vi "Save MC Test Data.vi"(5 "Initialise":bool, 6 "Stop":bool, 7 "Actual refresh rate (ms)":u32, 8 "error in (no error)":errorcluster, 9 "Initial Time Stamp":timestamp, 10 "Test Data In":dbl[][](array[numeric]), 11 "FPGA Ref in":T1) -> (0 "error out":errorcluster, 1 "MC state":enum16{"Waiting", "First frame", "Wrote Ref"}(ring), 2 "Test Data Out":dbl[][](array[numeric]), 4 "MC Data Save ON":bool)   [LabVIEW 2020]
uses:
  RIG-SPECIFIC FILES/FPGA Refs/FPGA Ref.ctl
  <vilib>/Utility/error.llb/Error Cluster From Error Code.vi
  <vilib>/rvi/errors/niLvFpgaAdjustHostInterfaceError.vi
  <vilib>/rvi/interface/nirviReadWriteControl/nirviReadWriteControl.xnode
  NiFpgaLv.dll
  <vilib>/rvi/interface/Simulation/niFpgaSimulationCallBeginRW.vi
panel:
  out "num_xyref_pixels":u16
  out "numxyzpixels":u16
  out "y_offset 3":fxp<+/-,16,8>
  out "X_Y_Z":bool[](array[boolean])
  out "MC state 2":enum16{"Waiting", "First frame", "Wrote Ref"}(ring)
  out "y_offset 2":fxp<+/-,16,8>
  out "y_offset":fxp<+/-,16,8>
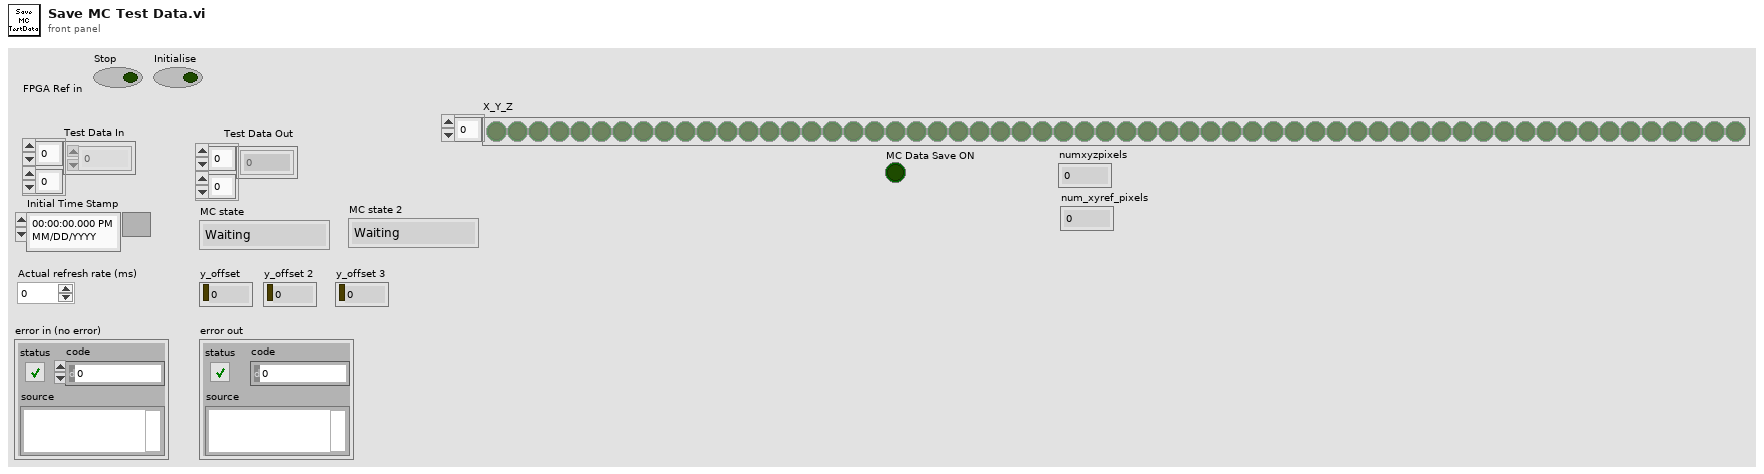
[diagram p1: front panel]
types:
  T1 = typedef "FPGA Ref.ctl" = refnum<k20>
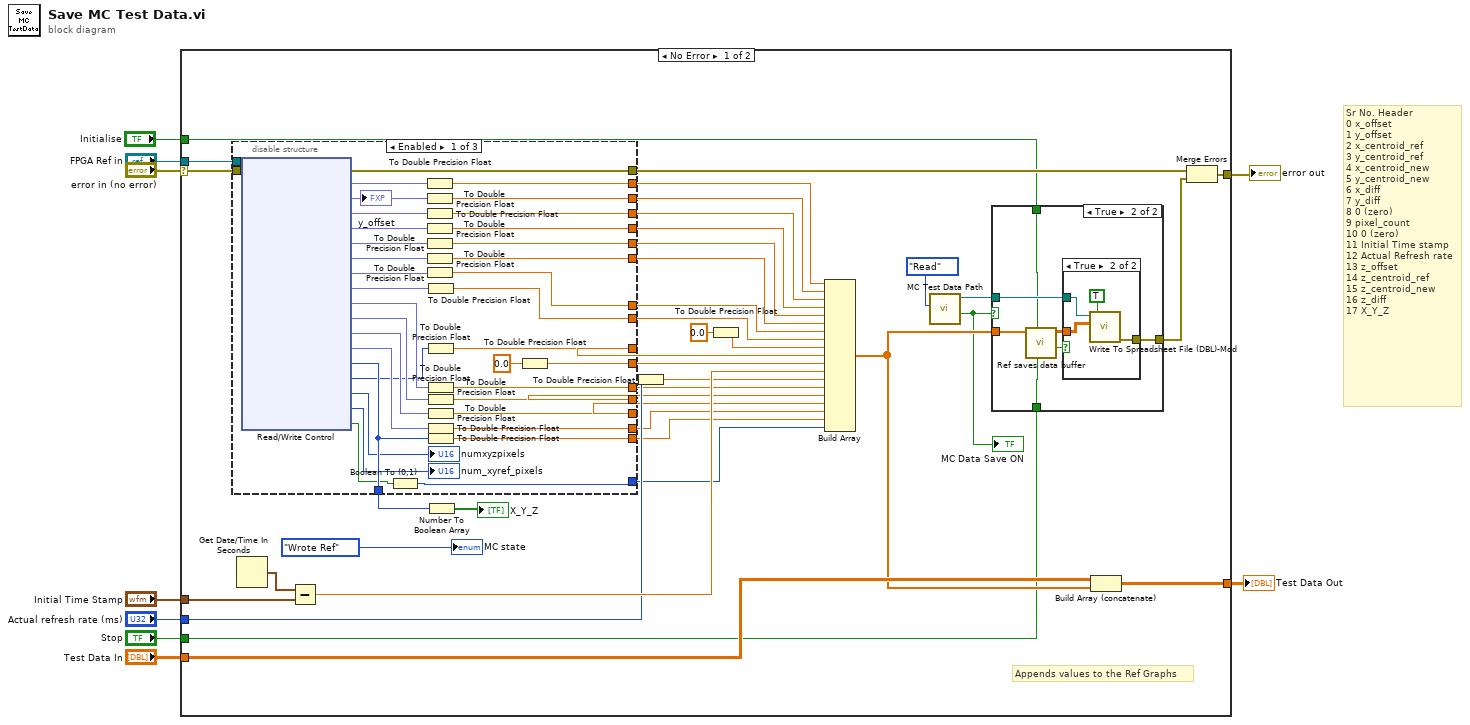
[diagram p0: block diagram]
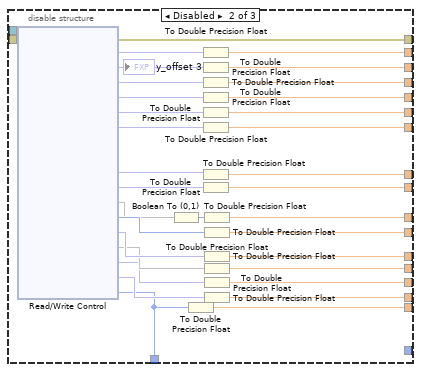
[diagram p2: hidden frame]
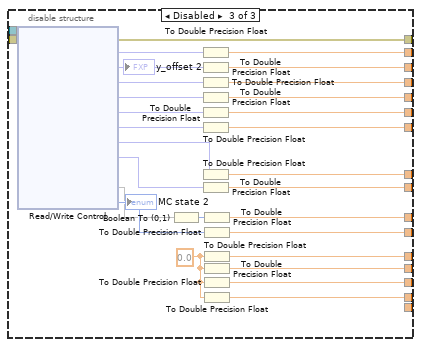
[diagram p3: hidden frame]
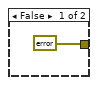
[diagram p4: hidden frame]
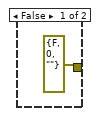
[diagram p5: hidden frame]
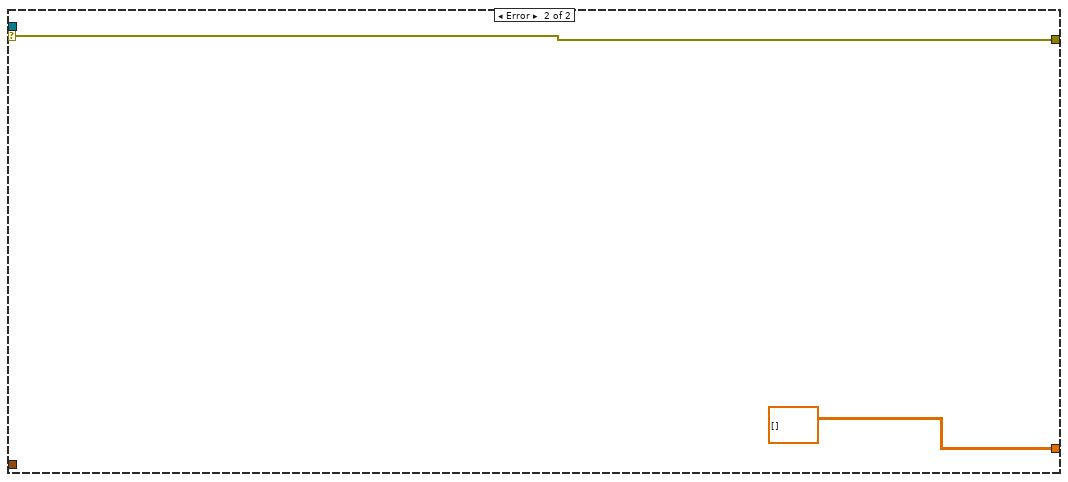
[diagram p6: hidden frame]
diagram:
  # "Sr No.\tHeader\n0\tx_offset\n1\ty_offset\n2\tx_centroid_ref\n3\ty_centroid_ref\n4\tx_centroid_new\n5\ty_centroid_new\n6\tx_diff\n7\ty_diff\n8\t0 (zero)\n9\tpixel_count\n10\t0 (zero)\n11\tInitial Time stamp\n12\tActual Refresh rate\n13\tz_offset\n14\tz_centroid_ref\n15\tz_centroid_new\n16\tz_diff\n17\tX_Y_Z"
  n1 = case shown="No Error" "error in (no error)" {
    selector: "error in (no error)" -> [w31 w163]
    tunnel: "FPGA Ref in" -> [w48 _]
    tunnel: "Test Data In" -> [w26 _]
    tunnel: "Initial Time Stamp" -> [w34 _]
    tunnel: [w32 dbl[][] []] -> w6
    tunnel: [w30 w163] -> w4
    tunnel: "Actual refresh rate (ms)" -> [w25 _]
    tunnel: "Stop" -> [w19 _]
    tunnel: "Initialise" -> [w24 _]
    frame No Error {
      # "Appends values to the Ref Graphs"
      n2 = disable-structure shown="Enabled" {
        disable-tunnel: w48 -> [w85 w119 w149]
        disable-tunnel: [w84 w117 w147] -> w47
        disable-tunnel: [w83 w116 w146] -> w46
        disable-tunnel: [w82 w113 w143] -> w44
        disable-tunnel: [w81 w112 w142] -> w43
        disable-tunnel: [w80 w111 w141] -> w42
        disable-tunnel: [w79 w110 w140] -> w41
        disable-tunnel: [w78 w109 w139] -> w40
        disable-tunnel: [w77 w108 w138] -> w39
        disable-tunnel: [w76 w107 w137] -> w38
        disable-tunnel: [w75 w106 w136] -> w37
        disable-tunnel: w31 -> [w66 w97 w126]
        disable-tunnel: [w65 w96 w125] -> w28
        disable-tunnel: [w52 w94 w124] -> w22
        disable-tunnel: [w60 w90 w123] -> w17
        disable-tunnel: [w59 w89 w122] -> w21
        disable-tunnel: [w58 w88 w121] -> w20
        disable-tunnel: [w57 w87 _] -> w16
        disable-tunnel: [w56 w86 _] -> w15
        disable-tunnel: [w49 _ _] -> w11
        frame Enabled {
          n3 = xnode "Read/Write Control"("FPGA VI Reference In"=w85, "error in"=w66) -> ("error out"=w65:errorcluster, "x_offset"=w73:fxp<+/-,16,8>, "y_offset"=w71:fxp<+/-,16,8>, "x_centroid_ref"=w67:fxp<+,32,16>, "y_centroid_ref"=w68:fxp<+,32,16>, "x_centroid_new"=w69:fxp<+,32,16>, "y_centroid_new"=w70:fxp<+,32,16>, "x_diff"=w72:fxp<+/-,16,8>, "y_diff"=w74:fxp<+/-,16,8>, "z offset"=w64:fxp<+/-,16,8>, "z_centroid_ref"=w63:fxp<+,32,16>, "z_centroid_new"=w61:fxp<+,32,16>, "z_diff"=w62:fxp<+/-,16,8>, "X_Y_Z"=w56:u64, "pixel_count"=w55:u16, "numxyzpixels"=→"numxyzpixels":u16, "num_xyref_pixels"=→"num_xyref_pixels":u16, "background_mc"=w50:bool)  [unwired: 1 out]
          "y_offset" <- w71
          n4 = Boolean To (0,1)(Boolean=w50) -> (0, 1=w49:i16)
          n5 = To Double Precision Float(number=w73) -> (double precision float=w82:dbl)
          n6 = To Double Precision Float(number=w71) -> (double precision float=w75:dbl)
          n7 = To Double Precision Float(number=w67) -> (double precision float=w76:dbl)
          n8 = To Double Precision Float(number=w68) -> (double precision float=w77:dbl)
          n9 = To Double Precision Float(number=w69) -> (double precision float=w78:dbl)
          n10 = To Double Precision Float(number=w70) -> (double precision float=w79:dbl)
          n11 = To Double Precision Float(number=w72) -> (double precision float=w80:dbl)
          n12 = To Double Precision Float(number=w74) -> (double precision float=w81:dbl)
          n13 = To Double Precision Float(number=w55) -> (double precision float=w83:dbl)
          n14 = To Double Precision Float(number=w64) -> (double precision float=w52:dbl)
          n15 = To Double Precision Float(number=w63) -> (double precision float=w60:dbl)
          n16 = To Double Precision Float(number=w61) -> (double precision float=w59:dbl)
          n17 = To Double Precision Float(number=w62) -> (double precision float=w58:dbl)
          n18 = To Double Precision Float(number=w56) -> (double precision float=w57:dbl)
          n19 = To Double Precision Float(number=0.0) -> (double precision float=w84:dbl)
        }
        frame Disabled {
          n20 = xnode "Read/Write Control"("FPGA VI Reference In"=w119, "error in"=w97) -> ("error out"=w96:errorcluster, "x_offset"=w104:fxp<+/-,16,8>, "y_offset"=w102:fxp<+/-,16,8>, "x_centroid_ref"=w98:fxp<+,32,16>, "y_centroid_ref"=w99:fxp<+,32,16>, "x_centroid_new"=w100:fxp<+,32,16>, "y_centroid_new"=w101:fxp<+,32,16>, "x_diff"=w103:fxp<+/-,16,8>, "y_diff"=w105:fxp<+/-,16,8>, "_SS"=w114, "Data Out"=w118:u64, "z offset"=w95:fxp<+/-,16,8>, "z_centroid_ref"=w93, "z_centroid_new"=w91:fxp<+,32,16>, "z_diff"=w92:fxp<+/-,16,8>, "X_Y_Z"=w86:u64)  [unwired: 3 out]
          "y_offset 3" <- w102
          n21 = Boolean To (0,1)(Boolean=w114) -> (0, 1=w115:i16)
          n22 = To Double Precision Float(number=w86) -> (double precision float=w87:dbl)
          n23 = To Double Precision Float(number=w104) -> (double precision float=w113:dbl)
          n24 = To Double Precision Float(number=w102) -> (double precision float=w106:dbl)
          n25 = To Double Precision Float(number=w98) -> (double precision float=w107:dbl)
          n26 = To Double Precision Float(number=w99) -> (double precision float=w108:dbl)
          n27 = To Double Precision Float(number=w100) -> (double precision float=w109:dbl)
          n28 = To Double Precision Float(number=w101) -> (double precision float=w110:dbl)
          n29 = To Double Precision Float(number=w103) -> (double precision float=w111:dbl)
          n30 = To Double Precision Float(number=w105) -> (double precision float=w112:dbl)
          n31 = To Double Precision Float(number=w115) -> (double precision float=w116:dbl)
          n32 = To Double Precision Float(number=w118) -> (double precision float=w117:dbl)
          n33 = To Double Precision Float(number=w95) -> (double precision float=w94:dbl)
          n34 = To Double Precision Float(number=w93) -> (double precision float=w90:dbl)
          n35 = To Double Precision Float(number=w91) -> (double precision float=w89:dbl)
          n36 = To Double Precision Float(number=w92) -> (double precision float=w88:dbl)
        }
        frame Disabled {
          w120 = 0.0
          n37 = xnode "Read/Write Control"("FPGA VI Reference In"=w149, "error in"=w126) -> ("error out"=w125:errorcluster, "x_offset"=w134:fxp<+/-,16,8>, "y_offset"=w132:fxp<+/-,16,8>, "x_centroid_ref"=w127:fxp<+,32,16>, "y_centroid_ref"=w128:fxp<+,32,16>, "x_centroid_new"=w129:fxp<+,32,16>, "y_centroid_new"=w130:fxp<+,32,16>, "x_diff"=w133:fxp<+/-,16,8>, "y_diff"=w135:fxp<+/-,16,8>, "MC State"=→"MC state 2", "_SS"=w144, "Data Out"=w148:u64)  [unwired: 1 out]
          "y_offset 2" <- w132
          n38 = Boolean To (0,1)(Boolean=w144) -> (0, 1=w145:i16)
          n39 = To Double Precision Float(number=w134) -> (double precision float=w143:dbl)
          n40 = To Double Precision Float(number=w132) -> (double precision float=w136:dbl)
          n41 = To Double Precision Float(number=w127) -> (double precision float=w137:dbl)
          n42 = To Double Precision Float(number=w128) -> (double precision float=w138:dbl)
          n43 = To Double Precision Float(number=w129) -> (double precision float=w139:dbl)
          n44 = To Double Precision Float(number=w130) -> (double precision float=w140:dbl)
          n45 = To Double Precision Float(number=w133) -> (double precision float=w141:dbl)
          n46 = To Double Precision Float(number=w135) -> (double precision float=w142:dbl)
          n47 = To Double Precision Float(number=w145) -> (double precision float=w146:dbl)
          n48 = To Double Precision Float(number=w148) -> (double precision float=w147:dbl)
          n49 = To Double Precision Float(number=w120) -> (double precision float=w124:dbl)
          n50 = To Double Precision Float(number=w120) -> (double precision float=w123:dbl)
          n51 = To Double Precision Float(number=w120) -> (double precision float=w122:dbl)
          n52 = To Double Precision Float(number=w120) -> (double precision float=w121:dbl)
        }
      }
      n53 = Get Date/Time In Seconds() -> (seconds since 1Jan1904=w18:timestamp)
      n54 = Subtract(x=w18, y=w34) -> (x-y=w33:dbl)
      n55 = Number To Boolean Array(number=w15) -> (Boolean array=→"X_Y_Z":bool[])
      n56 = To Double Precision Float(number=w25) -> (double precision float=w27:dbl)
      n57 = To Double Precision Float(number=0.0) -> (double precision float=w45:dbl)
      n58 = Build Array(w44, w37, w38, w39, w40, w41, w42, w43, w45, w46, w47, w33, w27, w22, w17, w21, w20, w16, w11) -> (w23:dbl[])
      n59 = call "MC Test Data Path.vi"("State"=enum16{"Initialise", "Write", "Read"}."Read") -> ("Save Test Data"=w10:bool, "Test GraphData Path"=w35:path)  [unwired: 8 in, 1 out]
      "MC Data Save ON" <- w10
      n60 = case shown="True" w10 {
        tunnel: w35 -> [_ w157]
        tunnel: [errorcluster {"status"=FALSE, "code"=0, "source"=""} ("error out") w156] -> w29
        tunnel: w23 -> [_ w155]
        tunnel: w24 -> [_ w153]
        tunnel: w19 -> [_ w152]
        frame False {
        }
        frame True {
          n61 = call "Ref saves data buffer.vi"("Stop"=w152, "Initialise"=w153, "Array in"=w155) -> ("Save data"=w151:bool, "Array out"=w154:dbl[][])  [unwired: 7 in]
          n62 = case shown="True" w151 {
            tunnel: w157 -> [_ w162]
            tunnel: [errorcluster {"status"=FALSE, "code"=0, "source"=""} ("error out") w160] -> w156
            tunnel: w154 -> [_ w159]
            frame False {
            }
            frame True {
              n63 = call <userlib>:"Write To Spreadsheet File (DBL)-Mod.vi"("append to file? (new file:F)"=TRUE, "2D data"=w159, "file path (dialog if empty)"=w162) -> ("error out"=w160:errorcluster)  [unwired: 7 in, 1 out]
            }
          }
        }
      }
      n64 = Build Array (concatenate)(w26, w23) -> (w32:dbl[][])
      n65 = Merge Errors(w28, w29) -> (w30:errorcluster)
      "MC state" <- enum16{"Waiting", "First frame", "Wrote Ref"}."Wrote Ref" ("MC state")
    }
    frame Error {
    }
  }
  "Test Data Out" <- w6
  "error out" <- w4
